vi "显示数据.vi"() -> ()   [LabVIEW 2011]
panel:
  in  "停止":bool
  out "波形图":waveform(dbl)[](graph)
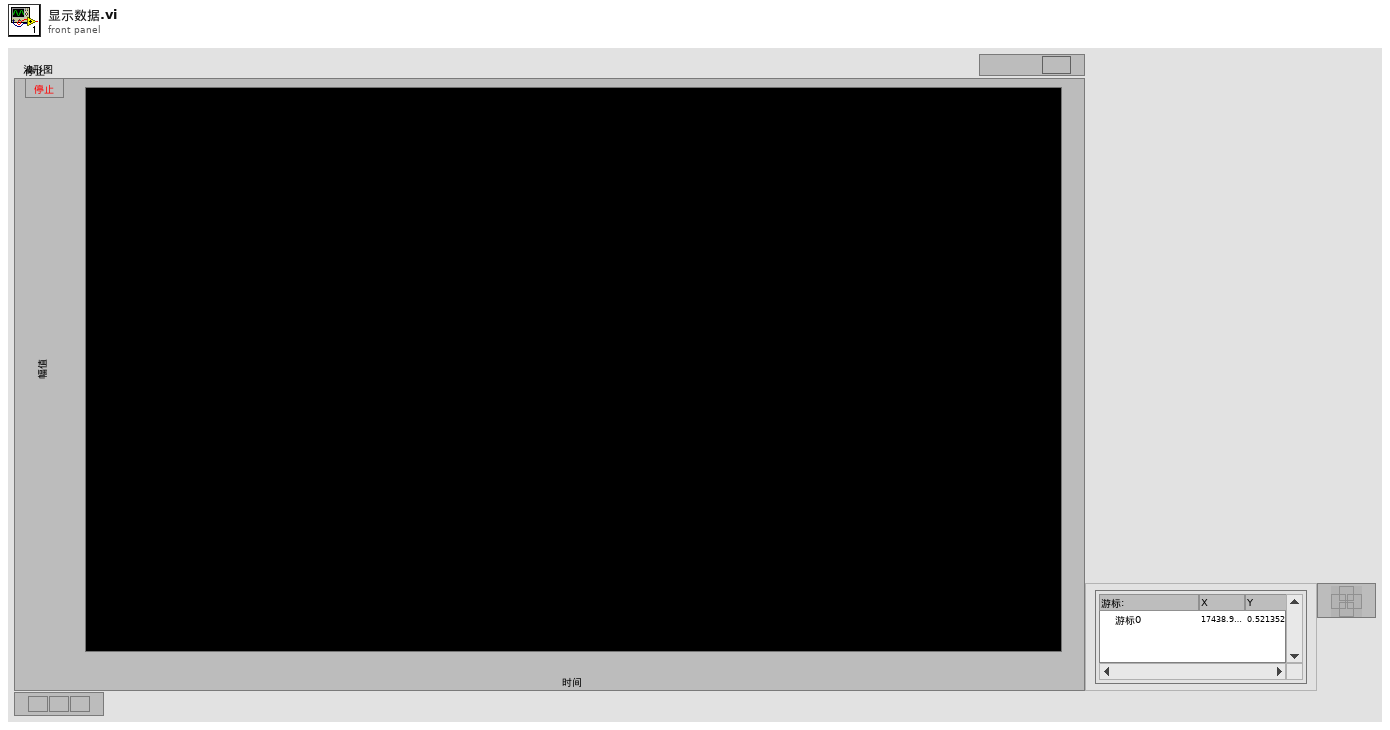
[diagram p1: front panel]
types:
  T1 = enum16{"open", "open or create", "create or replace", "create", "open (read-only)"}
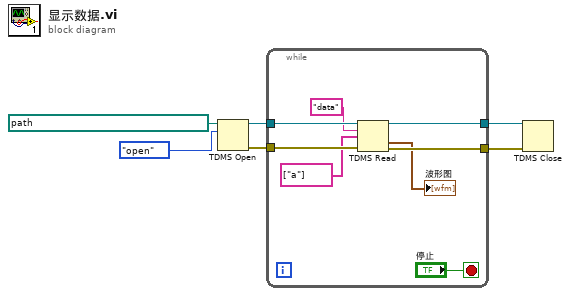
[diagram p0: block diagram]
diagram:
  n1 = TDMS Open(10:T1."open" ("操作(0:open)"), 11:path "E:/testdir/195-2/IV1/IV1-3.油压" ("文件路径")) -> (0:w3:errorcluster, 3:w6:refnum<k34>)  [unwired: 4 in]
  n2 = while {
    tunnel: w6 -> [w14]
    tunnel: w3 -> [w13]
    tunnel: [w10] -> w2
    tunnel: [w9] -> w1
    stop <- "停止" stop-if-true
    n3 = TDMS Read(0:w14, 5:"data" ("组名称输入"), 7:string[] ["a"] ("通道名输入"), 11:w13) -> (4:w10:refnum<k34>, 10:→"波形图":waveform(dbl)[], 15:w9:errorcluster)  [unwired: 4 in, 3 out]
  }
  n4 = TDMS Close(8:w1, 11:w2) -> ()  [unwired: 2 out]
